vi "bmlv_tests_dict_in_loops.vi"() -> ()   [LabVIEW 2014]
uses:
  bmlv/Dictionary/Dictionary.lvclass
panel:
  in  "Auto-Inc":bool
  in  "Initial value":dbl
  out "Variant":variant
  in  "Dump":bool
  in  "Write":bool
  in  "Name":string
  in  "Boolean":bool
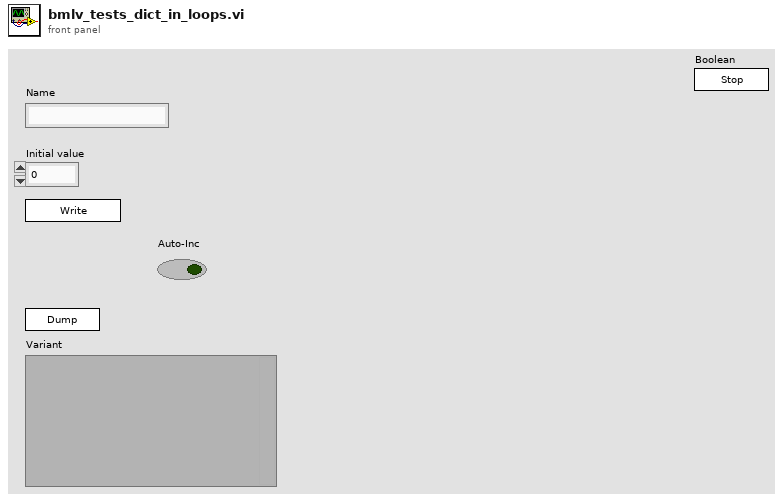
[diagram p1: front panel]
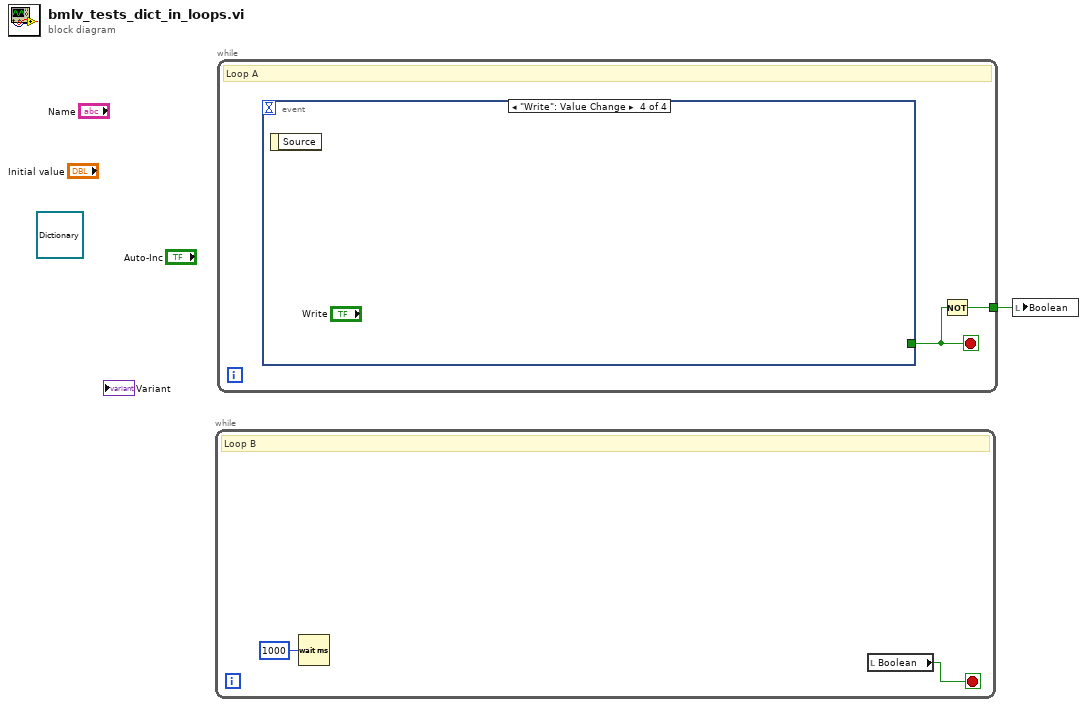
[diagram p0: block diagram]
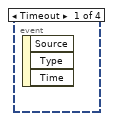
[diagram p2: hidden frame]
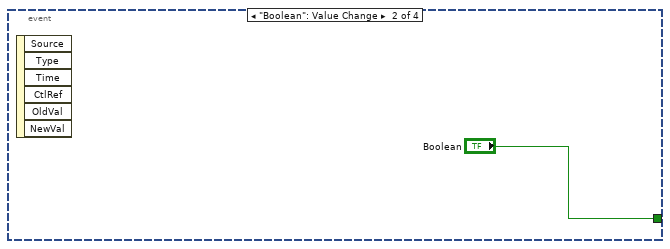
[diagram p3: hidden frame]
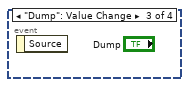
[diagram p4: hidden frame]
diagram:
  (unwired) refnum<class "Dictionary.lvclass"> refnum ("bmlv.lvlib:Dictionary.lvclass")
  n1 = while {
    stop <- w3 stop-if-true
    # "Loop B"
    n2 = Wait (ms)(milliseconds to wait=u32 1000) -> ()  [unwired: 1 out]
    n3 = local read "Boolean"() -> (w3:bool)
  }
  n4 = while {
    tunnel: [w4] -> w1
    stop <- w5 stop-if-true
    # "Loop A"
    n5 = event shown="[3] \"Write\": Value Change" {
      selector: _ -> [_ _ _ _]
      dyn-events: _ -> [_ _ _ _]
      timeout: _ -> [_ _ _ _]
      tunnel: [_ "Boolean" _ _] -> w5
      event Timeout {
        n6 = event-data() -> ()  [unwired: 1 in, 3 out]
      }
      event "Boolean": Value Change {
        n7 = event-data() -> ()  [unwired: 1 in, 6 out]
      }
      event "Dump": Value Change {
        n8 = event-data() -> ()  [unwired: 1 in, 1 out]
      }
      event "Write": Value Change {
        n9 = event-data() -> ()  [unwired: 1 in, 1 out]
      }
    }
    n10 = Not(x=w5) -> (.not. x?=w4:bool)
  }
  n11 = local write "Boolean"(w1) -> ()
